vi "FAMT View.vi"() -> ()   [LabVIEW 2015, in "FAMT Views.lvlib"]
uses:
  FAMT Views.lvlib
  Commands/Command Factory/Command Factory.lvclass
  User Events/User Events.lvclass
  User Events/User Events.lvclass/User Events.ctl
  Typedefs/Command Types.ctl
  Typedefs/State Types.ctl
  Typedefs/Actuator Types.ctl
  Translation Chart View.vi
  Moment Chart View.vi
  FC2 Chart View.vi
  Actuator Chart View.vi
  Typedefs/FAMT Typedefs.lvlib
  Controller/Controller.lvclass
  Settings/Settings.lvclass
panel:
  in  "Tab Control":T1(tab)
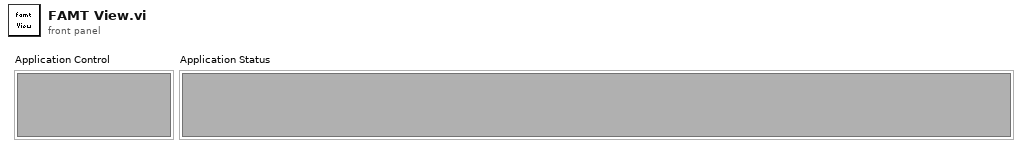
[diagram p1: front panel]
types:
  T1 = enum32{"Control", "Translation Chart", "Moment Chart", "Actuator Chart", "Cylinder Chart", "FC1 Chart", "FC2 Chart"}
  T2 = enum32{"invalid app kind", "Development System", "Run Time System", "Student Edition", "Embedded LabVIEW", "Evaluation", "Custom"}
  T3 = typedef "FAMT Typedefs.lvlib/Publish Data Events.ctl" = cluster{"State":refnum<user-event>, "ErrorCode":refnum<user-event>, "FC1 ILC Outputs":refnum<user-event>, "LogPath":refnum<user-event>, "FC1 ILC Inputs":refnum<user-event>, "Scan Progress":refnum<user-event>, "FC2 ILC Outputs":refnum<user-event>, "FC2 ILC Inputs":refnum<user-event>}
  T4 = typedef "FAMT Typedefs.lvlib/Subscribe Data Events.ctl" = cluster{"Command":refnum<user-event>}
  T5 = cluster{"Event Registration Refnum":refnum<event-registration>, "Event Registration Refnum":refnum<event-registration>, "Event Registration Refnum":refnum<event-registration>}
  T6 = typedef "FAMT Typedefs.lvlib/Command Types.ctl" = enum16{"Start", "Enable", "Disable", "Standby", "Shutdown", "Update"}
  T7 = typedef "FAMT Typedefs.lvlib/State Types.ctl" = enum16{"Offline State", "Fault State", "Standby State", "Disabled State", "Enabled State", "Wait For User Input State", "Perform Scan State"}
  T8 = typedef "FAMT Typedefs.lvlib/Actuator Types.ctl" = enum16{"Single", "Dual", "Dual Outer"}
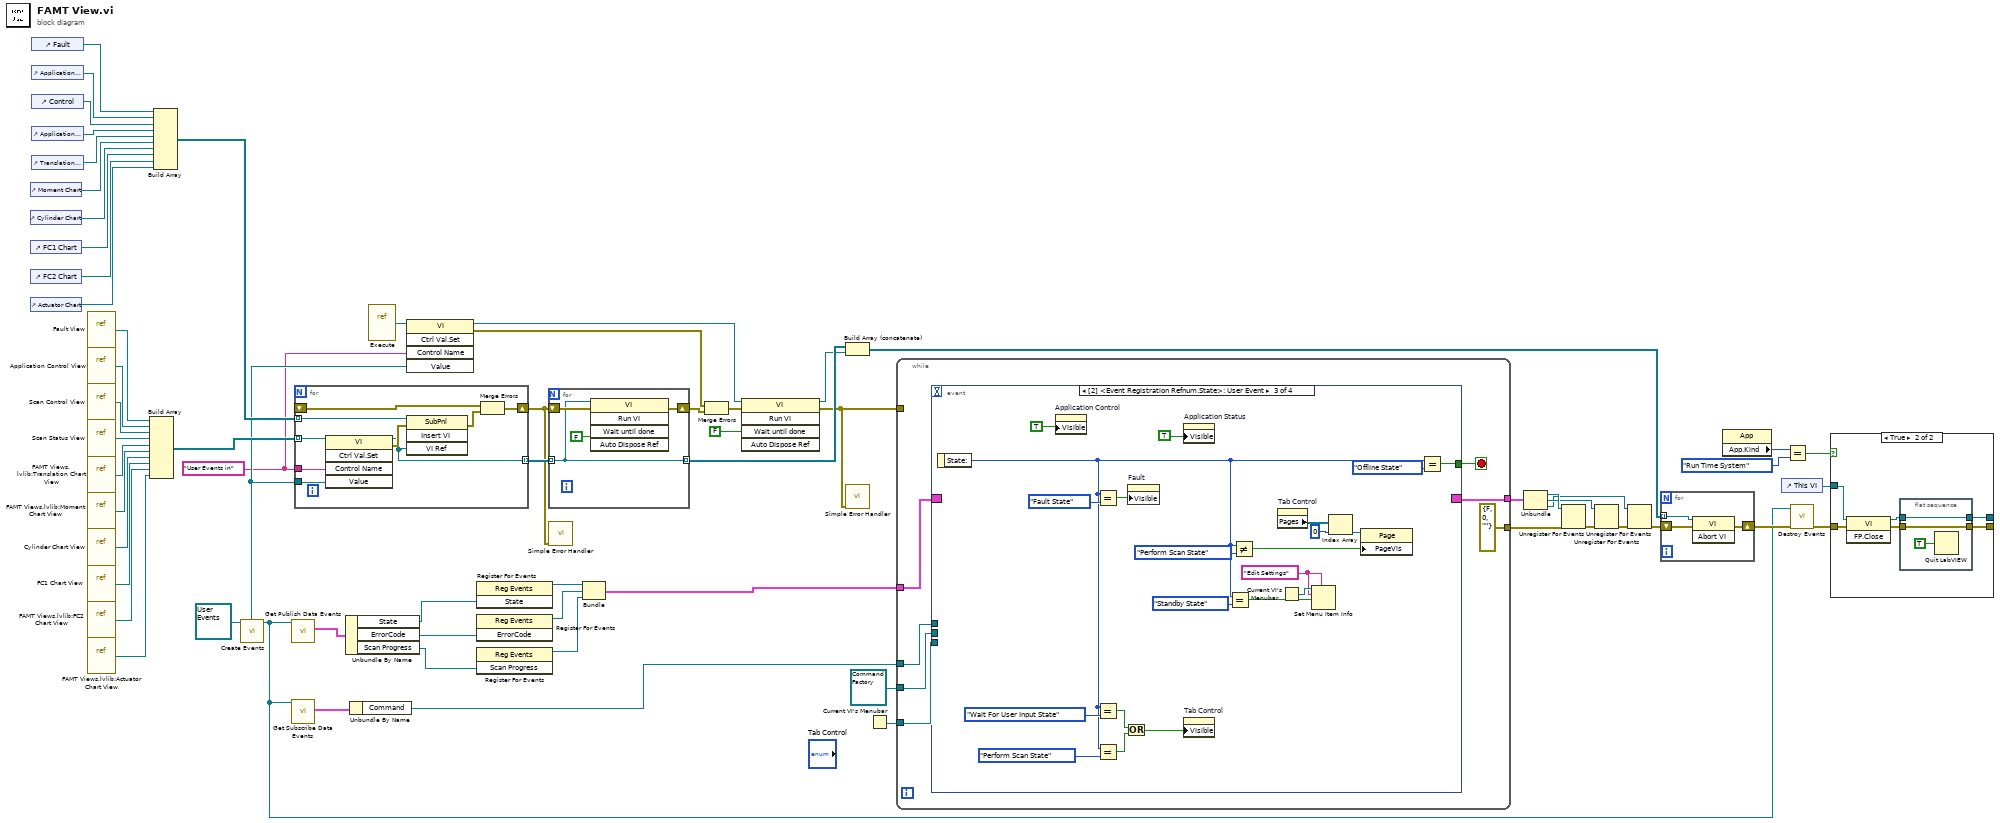
[diagram p0: block diagram]
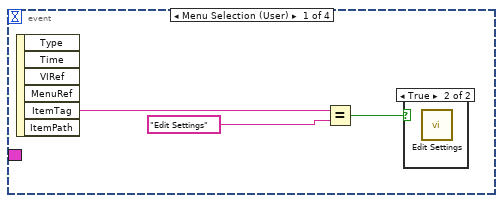
[diagram p3: hidden frame]
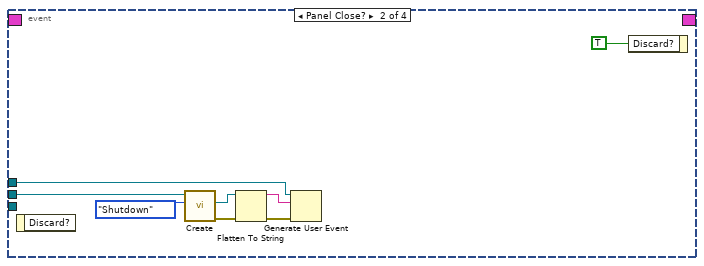
[diagram p5: hidden frame]
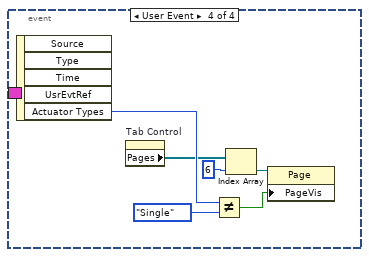
[diagram p6: hidden frame]
diagram:
  w33 = "User Events in" ("Control Name")
  n1 = control-ref of="Moment Chart"() -> (w15:refnum<vi>)
  n2 = control-ref of="Cylinder Chart"() -> (w14:refnum<vi>)
  n3 = control-ref of="FC1 Chart"() -> (w10:refnum<vi>)
  n4 = control-ref of="FC2 Chart"() -> (w8:refnum<vi>)
  n5 = control-ref of="Actuator Chart"() -> (w2:refnum<vi>)
  n6 = control-ref of="Fault"() -> (w22:refnum<vi>)
  n7 = control-ref of="Application Control"() -> (w21:refnum<vi>)
  n8 = control-ref of="Control"() -> (w20:refnum<vi>)
  n9 = control-ref of="Application Status"() -> (w19:refnum<vi>)
  n10 = control-ref of="Translation Chart"() -> (w18:refnum<vi>)
  n11 = vi-ref "Fault View.vi"() -> (w38:refnum<vi>)
  n12 = vi-ref "Application Control View.vi"() -> (w17:refnum<vi>)
  n13 = vi-ref "Scan Control View.vi"() -> (w16:refnum<vi>)
  n14 = vi-ref "Scan Status View.vi"() -> (w24:refnum<vi>)
  n15 = vi-ref "FAMT Views.lvlib:Translation Chart View.vi"() -> (w23:refnum<vi>)
  n16 = vi-ref "FAMT Views.lvlib:Moment Chart View.vi"() -> (w13:refnum<vi>)
  n17 = vi-ref "Cylinder Chart View.vi"() -> (w12:refnum<vi>)
  n18 = vi-ref "FC1 Chart View.vi"() -> (w11:refnum<vi>)
  n19 = vi-ref "FAMT Views.lvlib:FC2 Chart View.vi"() -> (w9:refnum<vi>)
  n20 = vi-ref "FAMT Views.lvlib:Actuator Chart View.vi"() -> (w1:refnum<vi>)
  n21 = Build Array(w38, w17, w16, w24, w23, w13, w12, w11, w9, w1) -> (w36:refnum<vi>[])
  n22 = Build Array(w22, w21, w20, w19, w18, w15, w14, w10, w8, w2) -> (w37:refnum<vi>[])
  n23 = call "Create Events.vi"("UserEvents in"=refnum<class "User Events.lvclass"> refnum) -> ("UserEvents out"=w34:refnum<class "User Events.lvclass">)  [unwired: 9 in, 1 out]
  n24 = call "Get Publish Data Events.vi"("UserEvents in"=w34) -> ("Publish Data Events"=w58:T3)  [unwired: 9 in, 1 out]
  n25 = call "Get Subscribe Data Events.vi"("UserEvents in"=w34) -> ("Subscribe Data Events"=w56:T4)  [unwired: 9 in, 1 out]
  n26 = for {
    tunnel: w34 -> [w72]
    tunnel: w37 -> [w71] mode=indexing
    tunnel: w36 -> [w65] mode=indexing
    shift-right: [w70] -> w26
    shift-left: _ -> [w69]
    tunnel: [w64] -> w35 mode=indexing
    tunnel: w33 -> [w68]
    n27 = invoke class="VI" method="Ctrl Val.Set"(reference=w65, "Control Name"=w68, "Value"=w72) -> (reference out=w64:refnum<vi>, error out=w67:errorcluster)  [unwired: 2 in, 3 out]
    n28 = invoke on="Invoke Node" class="SubPnl" method="Insert VI"(reference=w71, error in=w67, "VI Ref"=w64) -> (error out=w66:errorcluster)  [unwired: 1 in, 3 out]
    n29 = Merge Errors(w69, w66) -> (w70:errorcluster)
  }
  n30 = Unbundle By Name(w58) -> ("State"=w54:refnum<user-event>, "ErrorCode"=w52:refnum<user-event>, "Scan Progress"=w7:refnum<user-event>)
  n31 = Unbundle By Name(w56) -> ("Command"=w55:refnum<user-event>)
  n32 = vi-ref "Execute.vi"() -> (w49:refnum<vi>)
  n33 = invoke class="VI" method="Ctrl Val.Set"(reference=w49, "Control Name"=w33, "Value"=w34) -> (reference out=w48:refnum<vi>, error out=w30:errorcluster)  [unwired: 2 in, 3 out]
  n34 = register-events(w54) -> (reference out=w53:refnum<event-registration>)  [unwired: 2 in, 1 out]
  n35 = register-events(w52) -> (reference out=w51:refnum<event-registration>)  [unwired: 2 in, 1 out]
  n36 = register-events(w7) -> (reference out=w6:refnum<event-registration>)  [unwired: 2 in, 1 out]
  n37 = for {
    shift-right: [w76] -> w32
    shift-left: w26 -> [w75]
    tunnel: w35 -> [w73] mode=indexing
    tunnel: [w73] -> w29 mode=indexing
    n38 = invoke class="VI" method="Run VI"(reference=w73, error in=w75, "Wait until done"=FALSE ("Wait Until Done")) -> (error out=w76:errorcluster)  [unwired: 2 in, 4 out]
  }
  n39 = call <vilib>:"Simple Error Handler.vi"("error in (no error)"=w26) -> ()  [unwired: 4 in, 5 out]
  n40 = Bundle("Event Registration Refnum"=w53, "Event Registration Refnum"=w51, "Event Registration Refnum"=w6) -> (w46:T5)  [unwired: 1 in]
  n41 = Merge Errors(w30, w32) -> (w31:errorcluster)
  n42 = invoke class="VI" method="Run VI"(reference=w48, error in=w31, "Wait until done"=FALSE ("Wait Until Done")) -> (reference out=w28:refnum<vi>, error out=w25:errorcluster)  [unwired: 2 in, 3 out]
  n43 = Build Array (concatenate)(w29, w28) -> (w27:refnum<vi>[])
  n44 = call <vilib>:"Simple Error Handler.vi"("error in (no error)"=w25) -> ()  [unwired: 4 in, 5 out]
  n45 = Current VI's Menubar() -> (w59:refnum<k9>)
  n46 = while {
    tunnel: refnum<class "Command Factory.lvclass"> refnum ("CommandFactory.lvclass") -> [w80]
    tunnel: [errorcluster {"status"=FALSE, "code"=0, "source"=""} ("error out")] -> w47
    tunnel: w59 -> [w78]
    tunnel: w46 -> [w82]
    tunnel: w55 -> [w79]
    tunnel: [w77] -> w45
    tunnel: w25 -> [_]
    stop <- w81 stop-if-true
    n47 = event shown="[2] <Event Registration Refnum.State>: User Event" {
      selector: w82 -> [_ _ _ _]
      dyn-events: [_ _ _ _] -> w77
      timeout: _ -> [_ _ _ _]
      tunnel: [_ _ w114 _] -> w81
      tunnel: w80 -> [_ w91 _ _]
      tunnel: w79 -> [_ w88 _ _]
      tunnel: w78 -> [_ _ _ _]
      event Menu Selection (User) {
        n48 = event-data() -> ("ItemTag"=w84:string)  [unwired: 1 in, 5 out]
        n49 = Equal?(x=w84, y="Edit Settings") -> (x = y?=w86:bool)
        n50 = case shown="True" w86 {
          frame False {
          }
          frame True {
            n51 = call "Edit Settings.vi"() -> ()  [unwired: 10 in, 2 out]
          }
        }
      }
      event Panel Close? {
        n52 = event-data() -> ()  [unwired: 1 in, 1 out]
        n53 = call-dynamic "Create.vi"("Command Types"=Command_Types."Shutdown" ("Command"), "Command Factory in"=w91) -> ("error out"=w94:errorcluster, "Command"=w93:refnum<class "Command.lvclass">)  [unwired: 7 in, 1 out]
        n54 = Flatten To String(anything=w93, error in (no error)=w94) -> (data string=w89:string, error out=w90:errorcluster)  [unwired: 2 in, 1 out]
        n55 = Generate User Event(user event=w88, event data cluster=w89, error in=w90) -> ()  [unwired: 1 in, 2 out]
        n56 = event-data("Discard?"=TRUE) -> ()  [unwired: 1 in, 1 out]
      }
      event User Event {
        w105 = "Edit Settings" ("menu tag")
        n57 = event-data() -> ("State:"=w102:T7)  [unwired: 1 in]
        n58 = property on="Application Control" class="SubPnl"("Visible"=TRUE) -> ()  [unwired: 2 in, 2 out]
        n59 = Equal?(x=w102, y=State_Types."Fault State") -> (x = y?=w111:bool)
        n60 = Equal?(x=w102, y=State_Types."Wait For User Input State") -> (x = y?=w100:bool)
        n61 = Equal?(x=w102, y=State_Types."Perform Scan State") -> (x = y?=w101:bool)
        n62 = Or(x=w100, y=w101) -> (x .or. y?=w99:bool)
        n63 = property on="Fault" class="SubPnl"("Visible"=w111) -> ()  [unwired: 2 in, 2 out]
        n64 = property on="Application Status" class="SubPnl"("Visible"=TRUE) -> ()  [unwired: 2 in, 2 out]
        n65 = property on="Tab Control" class="TabCtl (strict)"("Visible"=w99) -> ()  [unwired: 2 in, 2 out]
        n66 = Equal?(x=w102, y=State_Types."Standby State") -> (x = y?=w106:bool)
        n67 = Not Equal?(x=w102, y=State_Types."Perform Scan State") -> (x != y?=w95:bool)
        n68 = property on="Tab Control" class="TabCtl (strict)"() -> ("Pages"=w98:refnum<vi>[])  [unwired: 2 in, 2 out]
        n69 = Current VI's Menubar() -> (w107:refnum<k9>)
        n70 = Set Menu Item Info(7:w105, 9:w106, 10:w105, 11:w107) -> ()  [unwired: 3 in, 2 out]
        n71 = Index Array(array=w98, index=0) -> (element=w97:refnum<vi>)
        n72 = property class="Page"(reference=w97, "PageVis"=w95) -> ()  [unwired: 1 in, 2 out]
        n73 = Equal?(x=w102, y=State_Types."Offline State") -> (x = y?=w114:bool)
      }
      event User Event {
        n74 = event-data() -> ("Actuator Types"=w121:T8)  [unwired: 1 in, 4 out]
        n75 = property on="Tab Control" class="TabCtl (strict)"() -> ("Pages"=w119:refnum<vi>[])  [unwired: 2 in, 2 out]
        n76 = Not Equal?(x=w121, y=Actuator_Types."Single") -> (x != y?=w116:bool)
        n77 = Index Array(array=w119, index=6) -> (element=w118:refnum<vi>)
        n78 = property class="Page"(reference=w118, "PageVis"=w116) -> ()  [unwired: 1 in, 2 out]
      }
    }
  }
  n79 = Unbundle(w45) -> ("Event Registration Refnum"=w44:refnum<event-registration>, "Event Registration Refnum"=w42:refnum<event-registration>, "Event Registration Refnum"=w5:refnum<event-registration>)
  n80 = Unregister For Events(event registration refnum=w44, error in=w47) -> (error out=w43:errorcluster)
  n81 = Unregister For Events(event registration refnum=w42, error in=w43) -> (error out=w4:errorcluster)
  n82 = Unregister For Events(event registration refnum=w5, error in=w4) -> (error out=w3:errorcluster)
  n83 = for {
    tunnel: w27 -> [w122] mode=indexing
    shift-right: [w123] -> w41
    shift-left: w3 -> [w124]
    n84 = invoke class="VI" method="Abort VI"(reference=w122, error in=w124) -> (error out=w123:errorcluster)  [unwired: 1 in, 2 out]
  }
  n85 = property class="App"() -> ("App.Kind"=w63:T2)  [unwired: 2 in, 2 out]
  n86 = control-ref of="This VI"() -> (w40:refnum<vi>)
  n87 = Equal?(x=w63, y=T2."Run Time System") -> (x = y?=w61:bool)
  n88 = call "Destroy Events.vi"("error in (no error)"=w41, "UserEvents in"=w34) -> ("error out"=w39:errorcluster)  [unwired: 8 in, 1 out]
  n89 = case shown="True" w61 {
    tunnel: w40 -> [w126 w132]
    tunnel: w39 -> [w125 w131]
    tunnel: [w126 w129] -> _
    tunnel: [w125 w127] -> _
    frame False {
    }
    frame True {
      n90 = invoke class="VI" method="FP.Close"(reference=w132, error in=w131) -> (reference out=w128:refnum<vi>, error out=w130:errorcluster)  [unwired: 1 in, 1 out]
      n91 = flat-sequence {
        tunnel: w130 -> [w133]
        tunnel: [w134] -> w129
        tunnel: w128 -> [w134]
        tunnel: [w133] -> w127
        frame #0 {
          n92 = Quit LabVIEW(quit? (T)=TRUE) -> ()
        }
      }
    }
  }
